vi "FindTANGOPort.vi"(2 "Fehler (Eingang, kein Fehler)":errorcluster) -> (0 "Fehler (Ausgang)":errorcluster, 1 "TangoCOMPort":string)   [LabVIEW 2018]
uses:
  <vilib>/Instr/_visa.llb/VISA Find Search Mode.ctl
panel:
  out "Array":string[](array[string])
  out "VISA-Ressourcenname":refnum<visa-resource-name>
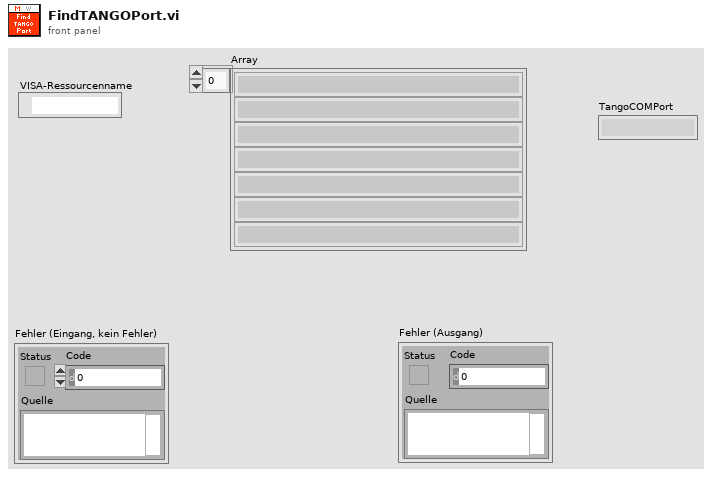
[diagram p1: front panel]
types:
  T1 = typedef "VISA Find Search Mode.ctl" = u32
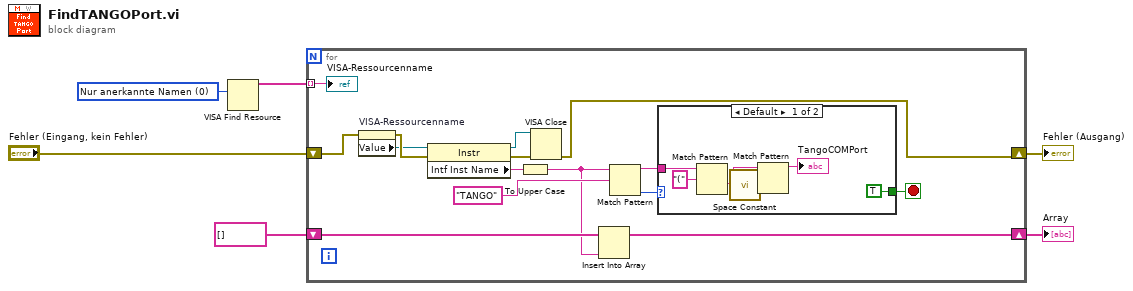
[diagram p0: block diagram]
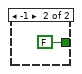
[diagram p2: hidden frame]
diagram:
  w6 = T1 0 items=["Nur anerkannte Namen"=0, "Nur Aliasnamen"=2, "Übereinstimmende Aliasnamen einschließen"=3, "Alle Aliasnamen einschließen"=4] ("Search Mode")
  n1 = VISA Find Resource(10:w6) -> (3:w5:string[])  [unwired: 2 in, 2 out]
  n2 = for {
    tunnel: w5 -> [w21] mode=indexing
    shift-right: [w18] -> w3
    shift-left: string[] [] -> [w20]
    shift-right: [w11] -> w2
    shift-left: "Fehler (Eingang, kein Fehler)" -> [w15]
    stop <- w9 stop-if-true
    n3 = property on="VISA-Ressourcenname" class="VISAName"(error in=w15) -> (error out=w19:errorcluster, "Value"=w14:refnum<visa-resource-name>)  [unwired: 1 in, 1 out]
    n4 = property class="Instr"(reference=w14, error in=w19) -> (reference out=w10:refnum<visa-resource-name>, error out=w12:errorcluster, "Intf Inst Name"=w8:string)
    n5 = To Upper Case(1:w8) -> (0:w7:string)
    n6 = VISA Close(VISA resource name=w10, error in (no error)=w12) -> (error out=w11:errorcluster)
    n7 = Insert Into Array(array=w20, new element=w7) -> (w18:string[])  [unwired: 1 in]
    n8 = Match Pattern(string=w7, regular expression="TANGO" ("Regulärer Ausdruck")) -> (before substring=w13:string, offset past match=w16:i32)  [unwired: 1 in, 2 out]
    n9 = case shown="Default" w16 {
      tunnel: w13 -> [w24 _]
      tunnel: [TRUE FALSE] -> w9
      frame Default {
        n10 = Match Pattern(string=w24, regular expression="(" ("Regulärer Ausdruck")) -> (after substring=w26:string)  [unwired: 1 in, 3 out]
        n11 = call <vilib>:"Space Constant.vi"() -> ("String"=w25:string)
        n12 = Match Pattern(string=w26, regular expression=w25) -> (before substring=→"TangoCOMPort":string)  [unwired: 1 in, 3 out]
      }
      frame -1 {
      }
    }
    "VISA-Ressourcenname" <- w21
  }
  "Array" <- w3
  "Fehler (Ausgang)" <- w2
